vi "Add Wheel ID.vi"(6 "Identifier":u32, 8 "error in (no error)":errorcluster, 11 "Item Ref in":T1=18446744073709551615 format="%.0x") -> (0 "error out":errorcluster, 3 "Item Ref out":T1=18446744073709551615 format="%.0x", 4 "WheelID":i32)   [LabVIEW 2023, in "Vires VTD System Explorer.lvlib"]
uses:
  Vires VTD System Explorer.lvlib
  <vilib>/NI VeriStand/Custom Device API/Custom Device Item Ref.ctl
  Shared/Constants.vi
  Shared/Vires VTD Shared.lvlib
  <vilib>/NI VeriStand/Custom Device API/Custom Device API.lvlib
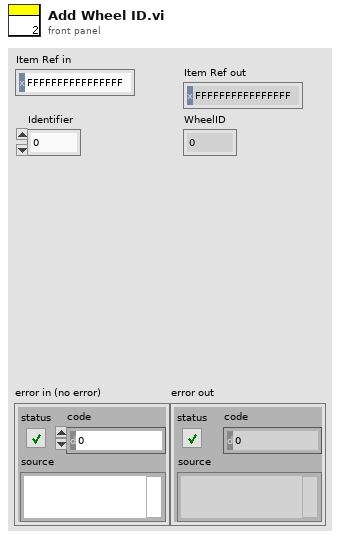
[diagram p1: front panel]
types:
  T1 = typedef "Custom Device API.lvlib/Custom Device Item Ref.ctl" = u64
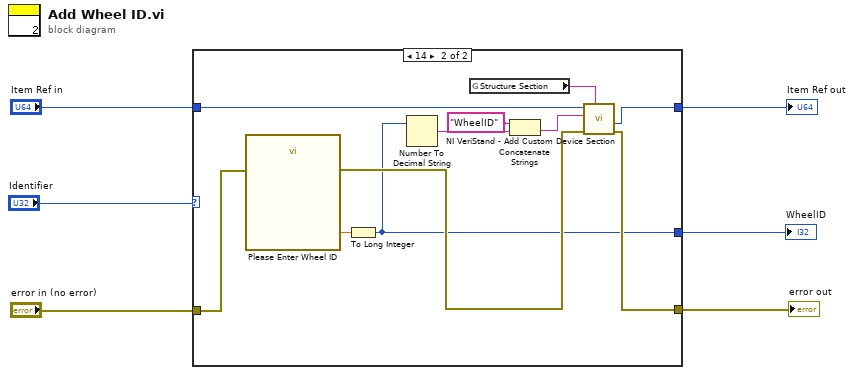
[diagram p0: block diagram]
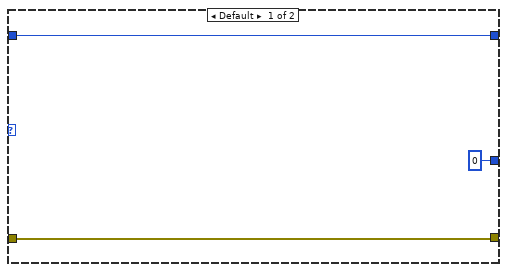
[diagram p2: hidden frame]
diagram:
  n1 = case shown="14" "Identifier" {
    tunnel: "Item Ref in" -> [w9 w19]
    tunnel: [w9 w18] -> w4
    tunnel: "error in (no error)" -> [w8 w16]
    tunnel: [w8 w17] -> w2
    tunnel: [0 w10] -> w1
    frame Default {
    }
    frame 14 {
      n2 = call "Please Enter Wheel ID"("error in (no error)"=w16) -> ("Wheel ID"=w11:dbl, "error out"=w15:errorcluster)  [unwired: 16 in, 1 out]
      n3 = To Long Integer(number=w11) -> (32bit integer=w10:i32)
      n4 = Number To Decimal String(number=w10) -> (decimal integer string=w13:string)  [unwired: 1 in]
      n5 = global read "Constants.vi" "Structure Section"() -> (w20:string)
      n6 = Concatenate Strings("WheelID" ("string"), w13) -> (w12:string)
      n7 = call <vilib>:"NI VeriStand - Add Custom Device Section.vi"("GUID (Default Section)"=w20, "error in (no error)"=w15, "Section Name"=w12, "Parent Ref in"=w19) -> ("error out"=w17:errorcluster, "Section Ptr"=w18:T1)  [unwired: 4 in, 2 out]
    }
  }
  "error out" <- w2
  "Item Ref out" <- w4
  "WheelID" <- w1
